vi "T90 Protokoll Textdatei.vi"() -> (3 "Textdatei":string[](array[string]))   [LabVIEW 2020, in "EPA 1065.lvlib" / "T90 Test 1065-308.lvlib"]
uses:
  T90 Test 1065-308.lvlib
  Seiten/FT-IR/FGV FT-IR Gasliste Aktionen.ctl
  Sprachverwaltung/FGV Aktion Tabelle zerlegen.ctl
  Aktion FGV T90.ctl
  Aktion FGV Datenmanagment.ctl
  Seiten/FT-IR/FT-IR.lvlib
  Sprachverwaltung/Sprachverwaltung.lvlib
  Seiten/System Einstellungen V2/System Einstellungen V2.lvlib
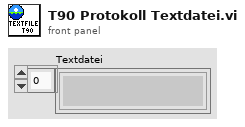
[diagram p1: front panel]
types:
  T1 = typedef "EPA 1065.lvlib/T90 Test 1065-308.lvlib/Aktion FGV Datenmanagment.ctl" = enum16{"init", "lesen", "Istwerte schreiben", "höchsten Peak setzen", "Auswerten", "Grenzen setzen", "Sollwert ändern", "Rise T10", "Rise T90", "Fall T90", "Fall T10", "Bit löschen", "Umschaltzeitpunkt"}
  T2 = typedef "EPA 1065.lvlib/T90 Test 1065-308.lvlib/Aktion FGV T90.ctl" = enum16{"lesen", "Konfig Daten", "speichern", "laden", "T90 aktiv", "T90 inaktiv", "Ext. Ventil aktivieren", "Ext. Ventil deaktivieren", "N2 spülen aktiv", "N2 spülen inaktiv", "Ergebnis Textfile"}
  T3 = typedef "Sprachverwaltung.lvlib/FGV Aktion Tabelle zerlegen.ctl" = enum16{"laden", "vereinzeln", "speichern"}
  T4 = typedef "FT-IR.lvlib/FGV FT-IR Gasliste Aktionen.ctl" = enum16{"lesen", "Gasliste FT-IR", "Gasliste ausgelesen", "laden", "speichern", "löschen"}
  T5 = typedef "EPA 1065.lvlib/T90 Test 1065-308.lvlib/T90 Konfig Daten.ctl" = cluster{"Bearbeiter:":string, "Komponente:":u16, "Gasflaschen Nr.:":string, "Accuracy":dbl, "Sollwert":dbl, "Modus":T6, "Abschaltzeit:":dbl, "Abweichung:":dbl, "Pfad:":path, "Textname:":string, "CG Aufschaltzeit:":dbl, "Einheit":string, "N2 Aufschaltzeit:":dbl, "Analysator":T7, "Gasflasche":T8, "Konfig Gasflasche":T9, "Frequency:":T10}
  T6 = typedef "EPA 1065.lvlib/T90 Test 1065-308.lvlib/Modus.ctl" = u16
  T7 = typedef "System Einstellungen V2.lvlib/Analysatoren.ctl" = string
  T8 = typedef "System Einstellungen V2.lvlib/Gasflasche Auswahl.ctl" = u16
  T9 = typedef "System Einstellungen V2.lvlib/Konfig Gasflasche.ctl" = bool
  T10 = typedef "EPA 1065.lvlib/T90 Test 1065-308.lvlib/Frequenz.ctl" = u16
  T11 = typedef "EPA 1065.lvlib/T90 Test 1065-308.lvlib/Result Textfile.ctl" = cluster{"Averaged T10-T90":string, "Averaged T90-T10":string, "Ergebnis x5 (T10 T90)":string, "Ergebnis x5 (T90 T10)":string, "Ergebnis 1":T12, "Ergebnis 2":T12, "Ergebnis 3":T12, "Ergebnis 4":T12}
  T12 = typedef "EPA 1065.lvlib/T90 Test 1065-308.lvlib/Ergebnis.ctl" = bool
  T13 = typedef "String - Ausgabefeld.ctl" = string
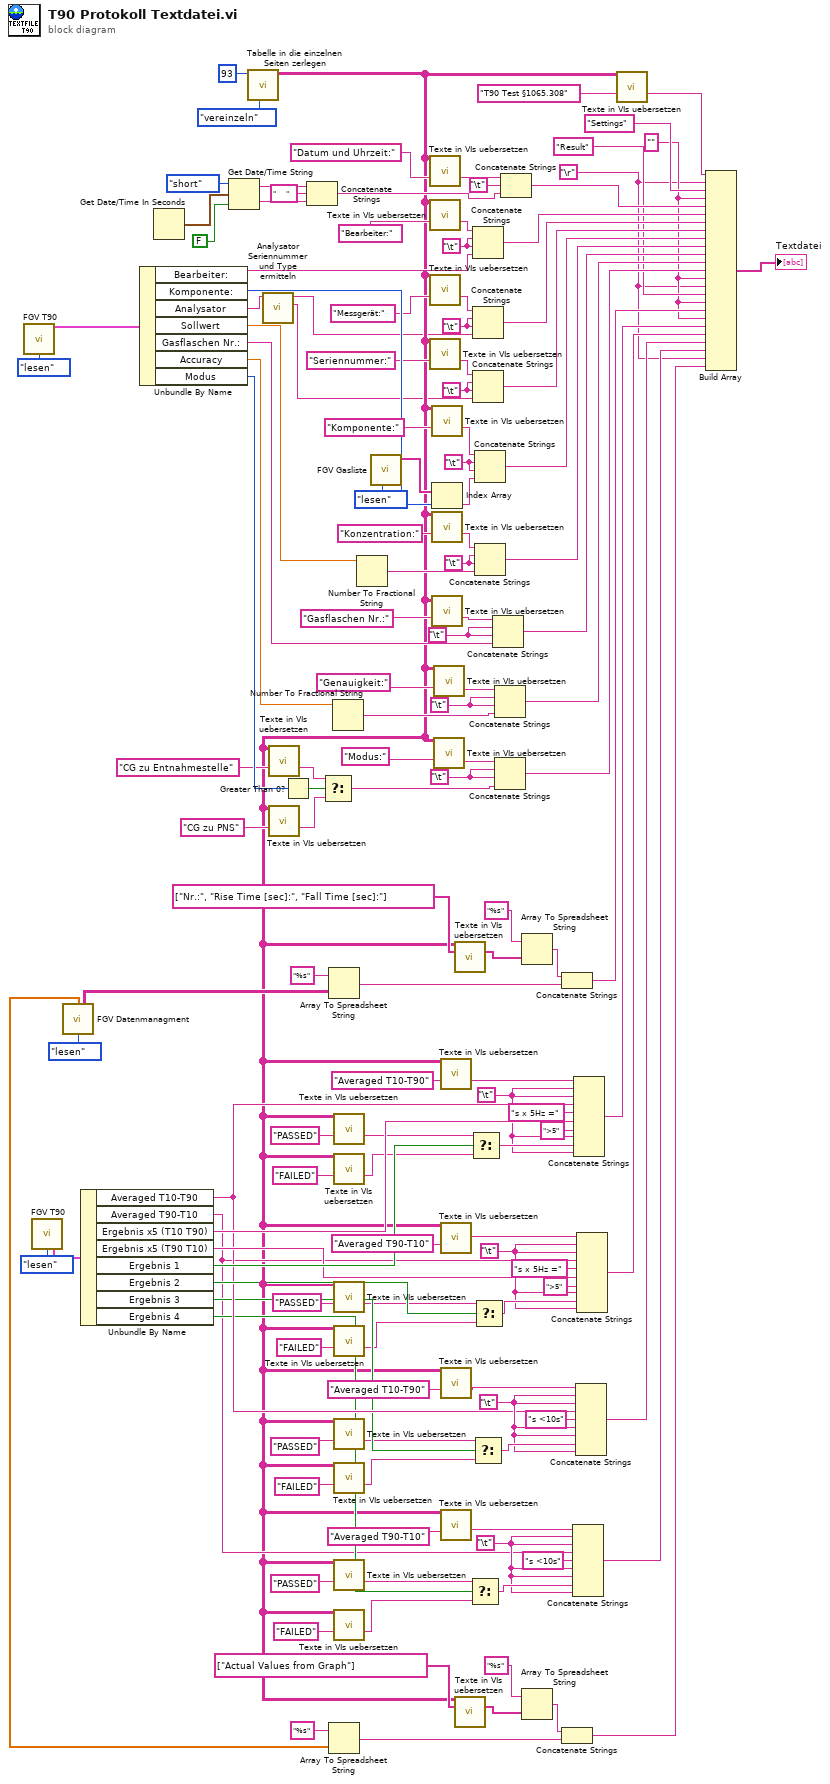
[diagram p0: block diagram]
diagram:
  w53 = "\t"
  w59 = "\t"
  w65 = "\t"
  w69 = "\t"
  w97 = "\t"
  w101 = "\t"
  w106 = "\t"
  w113 = "\t"
  w116 = "\t"
  w135 = "\t"
  w137 = "\t"
  w41 = "" ("Element")
  w142 = "\t"
  w6 = "\r"
  n1 = call "FGV T90.vi"("Aktion"=Aktion_FGV_T90."lesen") -> ("T90 Konfig Daten"=w85:T5)  [unwired: 9 in, 5 out]
  n2 = call "FGV T90.vi"("Aktion"=Aktion_FGV_T90."lesen") -> ("Result Textfile"=w76:T11)  [unwired: 9 in, 5 out]
  n3 = call "FGV Datenmanagment.vi"("Aktion"=Aktion_FGV_Datenmanagment."lesen") -> ("Aktuelle Messwerte"=w3:sgl[], "Ergebnistabelle"=w47:string[][])  [unwired: 7 in, 6 out]
  n4 = Unbundle By Name(w76) -> ("Averaged T10-T90"=w58:string, "Averaged T90-T10"=w50:string, "Ergebnis x5 (T10 T90)"=w74:string, "Ergebnis x5 (T90 T10)"=w62:string, "Ergebnis 1"=w71:T12, "Ergebnis 2"=w63:T12, "Ergebnis 3"=w56:T12, "Ergebnis 4"=w51:T12)
  n5 = Unbundle By Name(w85) -> ("Bearbeiter:"=w141:string, "Komponente:"=w138:u16, "Analysator"=w14:T7, "Sollwert"=w111:dbl, "Gasflaschen Nr.:"=w105:string, "Accuracy"=w98:dbl, "Modus"=w94:T6)
  n6 = Get Date/Time In Seconds() -> (seconds since 1Jan1904=w84:timestamp)
  n7 = Get Date/Time String(date format (0)=enum16{"short", "long", "abbreviated"}."short" ("Datumsformat (0)"), seconds (now)=w84, want seconds? (F)=FALSE ("Angabe von Sekunden? (F)")) -> (date string=w83:string, time string=w82:string)
  n8 = call "Tabelle in die einzelnen Seiten zerlegen.vi"("Aktion"=FGV_Aktion_Tabelle_zerlegen."vereinzeln", "Index (Seite)"=93) -> ("Sprachliste"=w7:string[][])  [unwired: 7 in, 2 out]
  n9 = call "Analysator Seriennummer und Type ermitteln.vi"("Analysator"=w14) -> ("Type"=w2:string, "Name für Protokoll"=w1:string)  [unwired: 8 in, 1 out]
  n10 = call "Texte in VIs uebersetzen.vi"("Sprachliste"=w7, "String zum Übersetzen"="CG zu Entnahmestelle") -> ("String zum Übersetzen"=w87:string)  [unwired: 9 in, 4 out]
  n11 = call "Texte in VIs uebersetzen.vi"("Sprachliste"=w7, "String zum Übersetzen"="CG zu PNS" ("f")) -> ("String zum Übersetzen"=w88:string)  [unwired: 9 in, 4 out]
  n12 = Greater Than 0?(x=w94) -> (x > 0?=w93:bool)
  n13 = Concatenate Strings(w83, "     " ("String"), w82) -> (w78:string)
  n14 = Select(t=w87, s=w93, f=w88) -> (s? t:f=w92:string)
  n15 = Array To Spreadsheet String(array=w47, 3:"%s" ("Format-String")) -> (spreadsheet string=w17:string)  [unwired: 1 in]
  n16 = Array To Spreadsheet String(array=w3, 3:"%s" ("Format-String")) -> (spreadsheet string=w11:string)  [unwired: 1 in]
  n17 = Number To Fractional String(number=w98) -> (F-format string=w99:string)  [unwired: 3 in]
  n18 = call "Texte in VIs uebersetzen.vi"("Sprachliste"=w7, "String zum Übersetzen"="PASSED" ("String")) -> ("String zum Übersetzen"=w36:string)  [unwired: 9 in, 4 out]
  n19 = call "Texte in VIs uebersetzen.vi"("Sprachliste"=w7, "String zum Übersetzen"="FAILED" ("f")) -> ("String zum Übersetzen"=w5:string)  [unwired: 9 in, 4 out]
  n20 = call "Texte in VIs uebersetzen.vi"("Sprachliste"=w7, "String zum Übersetzen"="PASSED" ("String")) -> ("String zum Übersetzen"=w23:string)  [unwired: 9 in, 4 out]
  n21 = call "Texte in VIs uebersetzen.vi"("Sprachliste"=w7, "String zum Übersetzen"="FAILED" ("f")) -> ("String zum Übersetzen"=w22:string)  [unwired: 9 in, 4 out]
  n22 = call "Texte in VIs uebersetzen.vi"("Sprachliste"=w7, "String zum Übersetzen"="PASSED" ("String")) -> ("String zum Übersetzen"=w25:string)  [unwired: 9 in, 4 out]
  n23 = call "Texte in VIs uebersetzen.vi"("Sprachliste"=w7, "String zum Übersetzen"="FAILED" ("f")) -> ("String zum Übersetzen"=w24:string)  [unwired: 9 in, 4 out]
  n24 = call "Texte in VIs uebersetzen.vi"("Sprachliste"=w7, "String zum Übersetzen"="PASSED" ("String")) -> ("String zum Übersetzen"=w27:string)  [unwired: 9 in, 4 out]
  n25 = call "Texte in VIs uebersetzen.vi"("Sprachliste"=w7, "String zum Übersetzen"="FAILED" ("f")) -> ("String zum Übersetzen"=w26:string)  [unwired: 9 in, 4 out]
  n26 = Number To Fractional String(number=w111) -> (F-format string=w110:string)  [unwired: 3 in]
  n27 = call "FGV Gasliste.vi"("Aktionen"=FGV_FT-IR_Gasliste_Aktionen."lesen") -> ("Aktuelle Gasliste FT-IR"=w139:T13[])  [unwired: 8 in, 2 out]
  n28 = call "Texte in VIs uebersetzen.vi"("Sprachliste"=w7, "String zum Übersetzen"="Datum und Uhrzeit:") -> ("String zum Übersetzen"=w128:string)  [unwired: 9 in, 4 out]
  n29 = call "Texte in VIs uebersetzen.vi"("Sprachliste"=w7, "String zum Übersetzen"="Bearbeiter:") -> ("String zum Übersetzen"=w126:string)  [unwired: 9 in, 4 out]
  n30 = call "Texte in VIs uebersetzen.vi"("Sprachliste"=w7, "String zum Übersetzen"="Messgerät:") -> ("String zum Übersetzen"=w124:string)  [unwired: 9 in, 4 out]
  n31 = call "Texte in VIs uebersetzen.vi"("Sprachliste"=w7, "String zum Übersetzen"="Seriennummer:") -> ("String zum Übersetzen"=w118:string)  [unwired: 9 in, 4 out]
  n32 = call "Texte in VIs uebersetzen.vi"("Sprachliste"=w7, "String zum Übersetzen"="Komponente:") -> ("String zum Übersetzen"=w122:string)  [unwired: 9 in, 4 out]
  n33 = Index Array(array=w139, index=w138) -> (element=w134:T13)
  n34 = call "Texte in VIs uebersetzen.vi"("Sprachliste"=w7, "String zum Übersetzen"="Konzentration:") -> ("String zum Übersetzen"=w114:string)  [unwired: 9 in, 4 out]
  n35 = call "Texte in VIs uebersetzen.vi"("Sprachliste"=w7, "String zum Übersetzen"="Gasflaschen Nr.:") -> ("String zum Übersetzen"=w108:string)  [unwired: 9 in, 4 out]
  n36 = call "Texte in VIs uebersetzen.vi"("Sprachliste"=w7, "String zum Übersetzen"="Genauigkeit:") -> ("String zum Übersetzen"=w103:string)  [unwired: 9 in, 4 out]
  n37 = call "Texte in VIs uebersetzen.vi"("Sprachliste"=w7, "String zum Übersetzen"="Modus:") -> ("String zum Übersetzen"=w96:string)  [unwired: 9 in, 4 out]
  n38 = call "Texte in VIs uebersetzen.vi"("Sprachliste"=w7, "String zum Übersetzen"="Averaged T10-T90") -> ("String zum Übersetzen"=w40:string)  [unwired: 9 in, 4 out]
  n39 = call "Texte in VIs uebersetzen.vi"("Sprachliste"=w7, "String zum Übersetzen"="Averaged T90-T10") -> ("String zum Übersetzen"=w35:string)  [unwired: 9 in, 4 out]
  n40 = call "Texte in VIs uebersetzen.vi"("Sprachliste"=w7, "String zum Übersetzen"="Averaged T10-T90") -> ("String zum Übersetzen"=w19:string)  [unwired: 9 in, 4 out]
  n41 = call "Texte in VIs uebersetzen.vi"("Sprachliste"=w7, "String zum Übersetzen"="Averaged T90-T10") -> ("String zum Übersetzen"=w18:string)  [unwired: 9 in, 4 out]
  n42 = call "Texte in VIs uebersetzen.vi"("Sprachliste"=w7, "String-Array zum Übersetzen"=string[] ["Nr.:", "Rise Time [sec]:", "Fall Time [sec]:"]) -> ("String-Array zum Übersetzen"=w15:string[])  [unwired: 9 in, 4 out]
  n43 = call "Texte in VIs uebersetzen.vi"("Sprachliste"=w7, "String-Array zum Übersetzen"=string[] ["Actual Values from Graph"]) -> ("String-Array zum Übersetzen"=w13:string[])  [unwired: 9 in, 4 out]
  n44 = Select(t=w27, s=w51, f=w26) -> (s? t:f=w54:string)
  n45 = Select(t=w36, s=w71, f=w5) -> (s? t:f=w70:string)
  n46 = Concatenate Strings(w126, w142, w142, w141) -> (w120:string)
  n47 = Concatenate Strings(w124, w137, w137, w1) -> (w136:string)
  n48 = Concatenate Strings(w118, w116, w116, w2) -> (w115:string)
  n49 = Select(t=w25, s=w56, f=w24) -> (s? t:f=w60:string)
  n50 = Select(t=w23, s=w63, f=w22) -> (s? t:f=w66:string)
  n51 = Concatenate Strings(w122, w135, w135, w134) -> (w119:string)
  n52 = Concatenate Strings(w114, w113, w113, w110) -> (w109:string)
  n53 = Concatenate Strings(w108, w106, w106, w105) -> (w104:string)
  n54 = Concatenate Strings(w103, w101, w101, w99) -> (w100:string)
  n55 = Concatenate Strings(w96, w97, w97, w92) -> (w91:string)
  n56 = Concatenate Strings(w128, "\t", w78) -> (w143:string)
  n57 = Array To Spreadsheet String(array=w15, 3:"%s" ("Format-String")) -> (spreadsheet string=w45:string)  [unwired: 1 in]
  n58 = Array To Spreadsheet String(array=w13, 3:"%s" ("Format-String")) -> (spreadsheet string=w10:string)  [unwired: 1 in]
  n59 = Concatenate Strings(w45, w17) -> (w42:string)
  n60 = Concatenate Strings(w10, w11) -> (w4:string)
  n61 = Concatenate Strings(w18, w53, w53, w50, "s <10s" ("String"), w53, w53, w54, w53) -> (w52:string)
  n62 = Concatenate Strings(w40, w69, w69, w58, "s x 5Hz =" ("String"), w74, ">5" ("String"), w69, w70, w69) -> (w73:string)
  n63 = Concatenate Strings(w19, w59, w59, w58, "s <10s" ("String"), w59, w59, w60, w59) -> (w57:string)
  n64 = Concatenate Strings(w35, w65, w65, w50, "s x 5Hz =" ("String"), w62, ">5" ("String"), w65, w66, w65) -> (w64:string)
  n65 = call "Texte in VIs uebersetzen.vi"("Sprachliste"=w7, "String zum Übersetzen"="T90 Test §1065.308") -> ("String zum Übersetzen"=w130:string)  [unwired: 9 in, 4 out]
  n66 = Build Array(w130, w6, "Settings" ("Element"), w41, w143, w120, w136, w115, w119, w109, w104, w100, w91, w41, w6, "Result" ("Element"), w41, w42, w41, w73, w64, w57, w52, w6, w4) -> (→"Textdatei":string[])
